vi "DSF.Engine.Runtime.Framework.Initialize Sequencer.vi"(8 "error in (no error)":errorcluster, 11 "Framework Runtime in":refnum<class "DSF.Engine.Runtime.Framework.lvclass">) -> (0 "error out":errorcluster, 3 "Framework Runtime out":refnum<class "DSF.Engine.Runtime.Framework.lvclass">)   [LabVIEW 2016, in "DSF.Engine.lvlib" / "DSF.Engine.Runtime.Framework.lvclass"]
uses:
  DSF.Engine.Runtime.Framework.lvclass
  DSF.Engine.Runtime.Framework.lvclass/DSF.Engine.Runtime.Framework.ctl
  Sequencer/DSF.Engine.Sequencer.lvclass
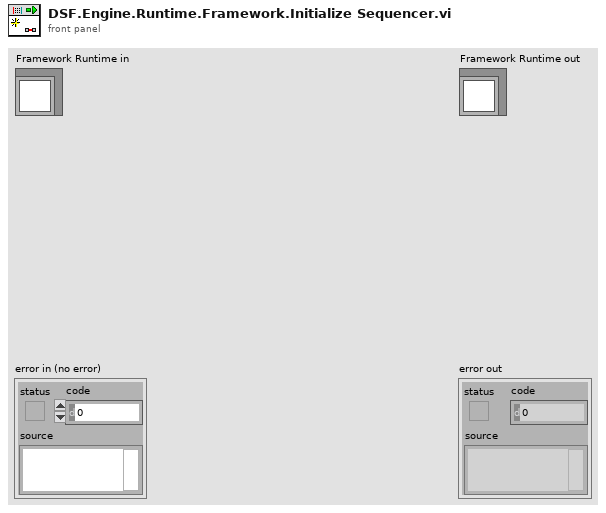
[diagram p1: front panel]
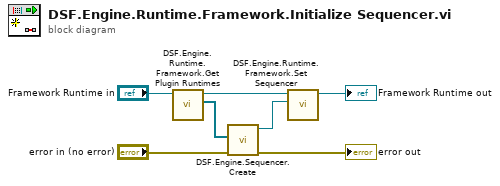
[diagram p0: block diagram]
diagram:
  n1 = call "DSF.Engine.Runtime.Framework.Get Plugin Runtimes.vi"("Framework Runtime in"="Framework Runtime in") -> ("Plugin Runtimes"=w6:refnum<class "DSF.Engine.Runtime.Plugin.lvclass">[], "Framework Runtime out"=w4:refnum<class "DSF.Engine.Runtime.Framework.lvclass">)  [unwired: 9 in]
  n2 = call "DSF.Engine.Sequencer.Create.vi"("error in (no error)"="error in (no error)", "Plugin Runtimes"=w6) -> ("error out"=→"error out":errorcluster, "Sequencer"=w5:refnum<class "DSF.Engine.Sequencer.lvclass">)  [unwired: 8 in]
  n3 = call "DSF.Engine.Runtime.Framework.Set Sequencer.vi"("Sequencer"=w5, "Framework Runtime in"=w4) -> ("Framework Runtime out"=→"Framework Runtime out":refnum<class "DSF.Engine.Runtime.Framework.lvclass">)  [unwired: 8 in, 1 out]
